vi "USB2XXXSPIW25Q32.vi"() -> ()   [LabVIEW 2010]
uses:
  PublicFiles/usb_device/USB2XXX.dll
panel:
  in  "pConfig":T1
  out "Read Data(Hex)":string
  in  "Read Data Count":i32=8
  in  "Start Addr(Hex)":u32 format="%x"
  in  "Write Data(Hex)":string="11 22 33 44 55 66 77 88"
  in  "Channel Index":i32(ring) items=["SPI1_CS0", "SPI2_CS0"]
  in  "Device Index":i32(ring) items=["0", "1", "2", "3", "4", "5"]
  out "Flag(T:Write;F:Read)":bool=TRUE
  in  "stop":bool
  in  "Read":bool
  in  "Write":bool
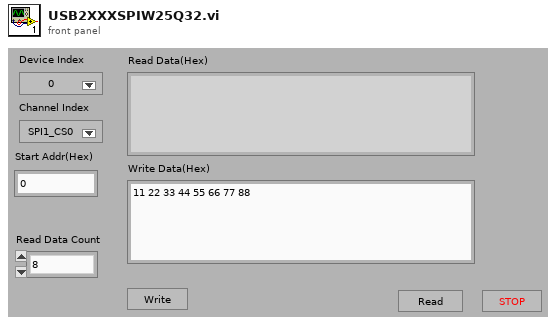
[diagram p1: front panel]
types:
  T1 = cluster{"Mode":i8, "Master":i8, "CPOL":i8, "CPHA":i8, "LSBFirst":i8, "SelPolarity":i8, "@dummy control@":i8, "@dummy control@":i8, "ClockSpeedHz":u32}
  T2 = enum16{"Init", "Write", "Read", "Idel", "Close", "Erase"}
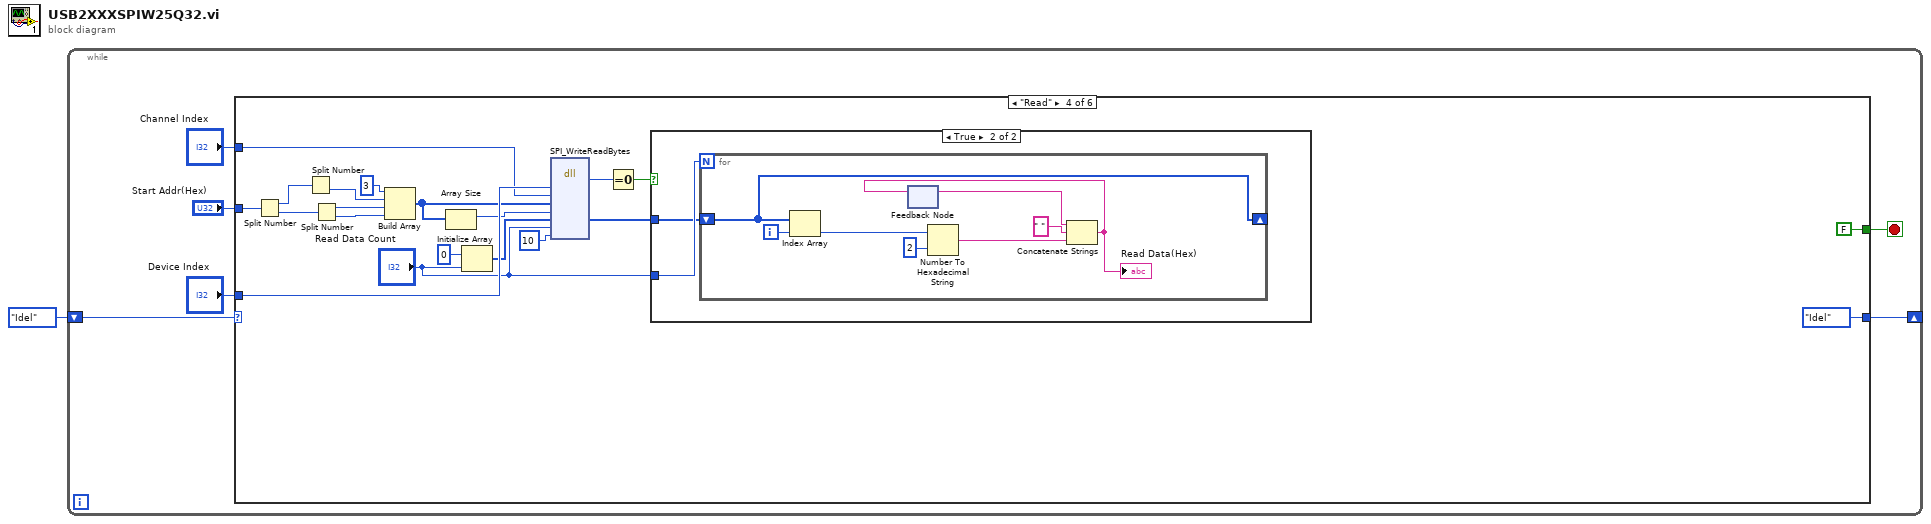
[diagram p0: block diagram]
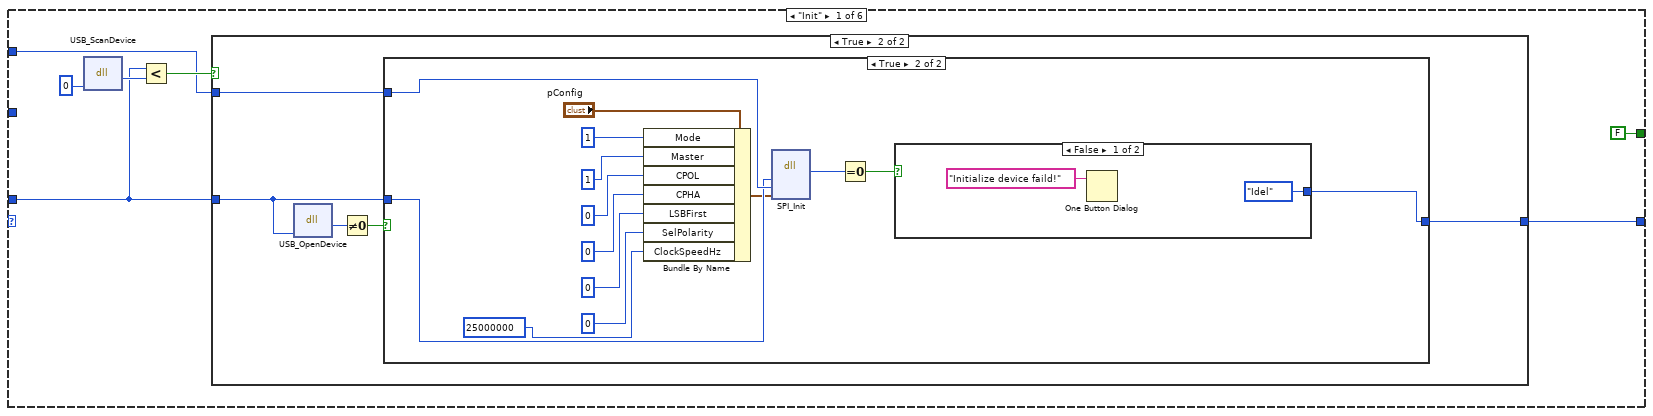
[diagram p2: hidden frame]
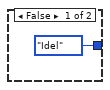
[diagram p3: hidden frame]
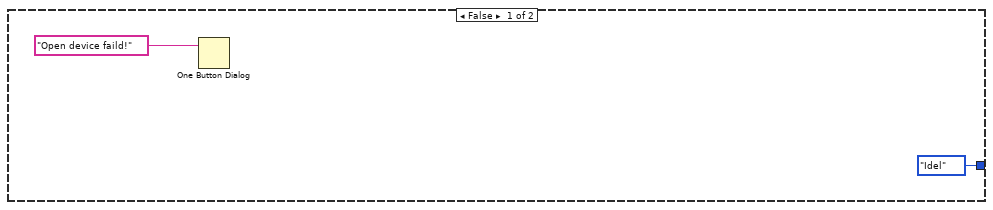
[diagram p4: hidden frame]
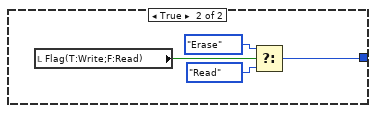
[diagram p5: hidden frame]
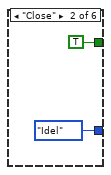
[diagram p6: hidden frame]
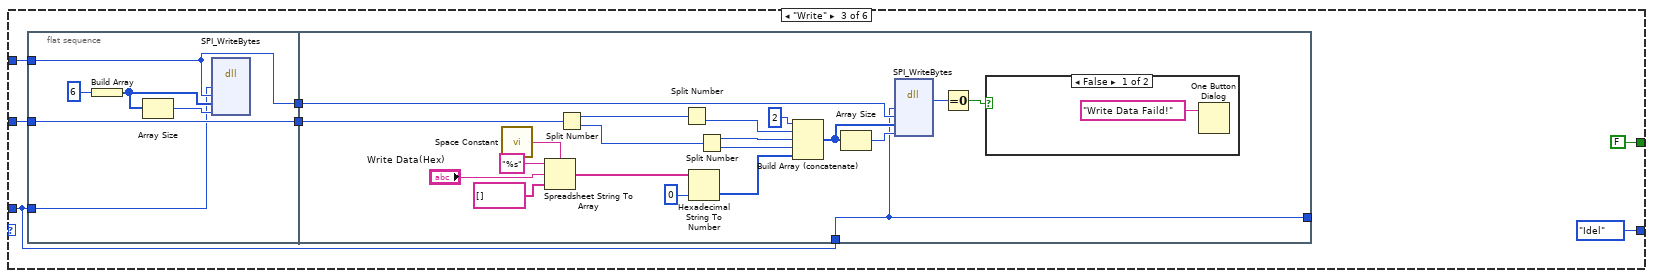
[diagram p7: hidden frame]
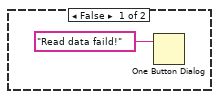
[diagram p9: hidden frame]
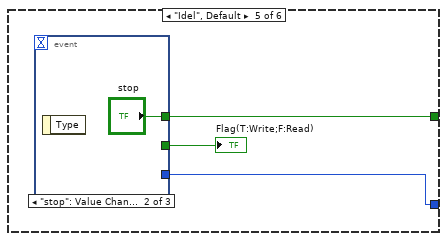
[diagram p10: hidden frame]
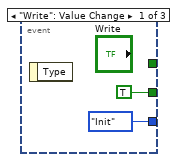
[diagram p11: hidden frame]
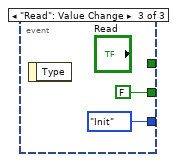
[diagram p12: hidden frame]
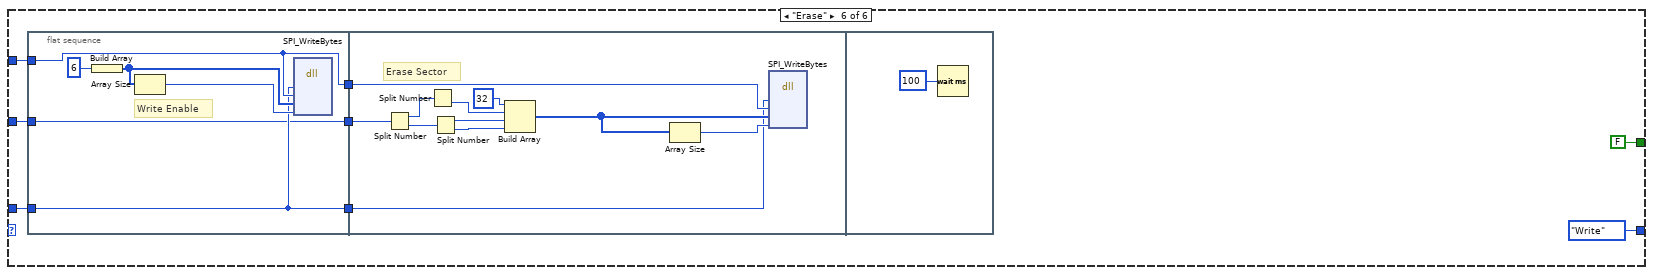
[diagram p13: hidden frame]
diagram:
  n1 = while {
    shift-right: [w6] -> _
    shift-left: T2."Idel" ("Enum") -> [w7]
    stop <- w2 stop-if-true
    n2 = case shown="\"Read\"" w7 {
      tunnel: [w11 T2."Idel" ("Enum") T2."Idel" ("Enum") T2."Idel" ("Enum") w110 T2."Write" ("Enum")] -> w6
      tunnel: "Device Index" -> [w8 _ w45 w87 _ w124]
      tunnel: "Channel Index" -> [w10 _ w50 w86 _ w123]
      tunnel: "Start Addr(Hex)" -> [_ _ w49 w89 _ w120]
      tunnel: [FALSE TRUE FALSE FALSE w111 FALSE] -> w2
      frame "Init" {
        n3 = dll-call lib="F:/OtherWork/STM32/USB2XXX_Example/trunk/Labview/PublicFiles/usb_device/USB2XXX.*" fn="USB_ScanDevice"("pDevNum"=0) -> (w13:i32)  [unwired: 4 in, 2 out]
        n4 = Less?(x=w8, y=w13) -> (x < y?=w12:bool)
        n5 = case shown="True" w12 {
          tunnel: w8 -> [_ w16]
          tunnel: w10 -> [_ w18]
          tunnel: [T2."Idel" ("Enum") w17] -> w11
          frame False {
          }
          frame True {
            n6 = dll-call lib="F:/OtherWork/STM32/USB2XXX_Example/trunk/Labview/PublicFiles/usb_device/USB2XXX.*" fn="USB_OpenDevice"("DevIndex"=w16) -> (w20:u8)  [unwired: 4 in, 2 out]
            n7 = Not Equal To 0?(x=w20) -> (x != 0?=w19:bool)
            n8 = case shown="True" w19 {
              tunnel: w18 -> [_ w34]
              tunnel: w16 -> [_ w33]
              tunnel: [T2."Idel" ("Enum") w35] -> w17
              frame False {
                n9 = One Button Dialog(message="Open device faild!") -> ()  [unwired: 1 in, 1 out]
              }
              frame True {
                n10 = Bundle By Name(cluster="pConfig", "Mode"=i8 1, "Master"=i8 1, "CPOL"=i8 0, "CPHA"=i8 0, "LSBFirst"=i8 0, "SelPolarity"=i8 0, "ClockSpeedHz"=u32 25000000) -> (w32:T1)
                n11 = dll-call lib="F:/OtherWork/STM32/USB2XXX_Example/trunk/Labview/PublicFiles/usb_device/USB2XXX.*" fn="SPI_Init"("DevIndex"=w33, "SPIIndex"=w34, "pConfig"=w32) -> (w31:i32)  [unwired: 6 in, 2 out]
                n12 = Equal To 0?(x=w31) -> (x = 0?=w36:bool)
                n13 = case shown="False" w36 {
                  tunnel: [T2."Idel" ("Enum") w41] -> w35
                  frame False {
                    n14 = One Button Dialog(message="Initialize device faild!") -> ()  [unwired: 1 in, 1 out]
                  }
                  frame True {
                    n15 = local read "Flag(T:Write;F:Read)"() -> (w42:bool)
                    n16 = Select(t=T2."Erase" ("Enum"), s=w42, f=T2."Read" ("Enum")) -> (s? t:f=w41:T2)
                  }
                }
              }
            }
          }
        }
      }
      frame "Close" {
      }
      frame "Write" {
        n17 = flat-sequence {
          tunnel: w45 -> [w52]
          tunnel: w50 -> [w53]
          tunnel: w49 -> [w54]
          tunnel: [w54] -> w48
          tunnel: [w53] -> w47
          tunnel: w48 -> [w60]
          tunnel: w47 -> [w59]
          tunnel: [w58] -> _
          tunnel: w45 -> [w58]
          frame #0 {
            n18 = Build Array(u8 6) -> (w56:u8[])
            n19 = Array Size(array=w56) -> (size(s)=w55:i32)
            n20 = dll-call lib="F:/OtherWork/STM32/USB2XXX_Example/trunk/Labview/PublicFiles/usb_device/USB2XXX.*" fn="SPI_WriteBytes"("DevIndex"=w52, "SPIIndex"=w53, "pWriteData"=w56, "WriteLen"=w55) -> ()  [unwired: 8 in, 2 out]
          }
          frame #1 {
            n21 = call <vilib>:"Space Constant.vi"() -> ("String"=w65:string)
            n22 = Spreadsheet String To Array(delimiter (Tab)=w65, format string="%s", spreadsheet string="Write Data(Hex)", array type (2D Dbl)=string[] []) -> (array=w62:string[])
            n23 = Split Number(x=w60) -> (hi(x)=w69:u16, lo(x)=w70:u16)
            n24 = Split Number(x=w69) -> (lo(x)=w71:u8)  [unwired: 1 out]
            n25 = Hexadecimal String To Number(string=w62, default (0uL)=u8 0 ("default (0 U32)")) -> (number=w74:u8[])  [unwired: 1 in, 1 out]
            n26 = Split Number(x=w70) -> (hi(x)=w72:u8, lo(x)=w73:u8)
            n27 = Build Array (concatenate)(u8 2, w71, w72, w73, w74) -> (w77:u8[])
            n28 = Array Size(array=w77) -> (size(s)=w75:i32)
            n29 = dll-call lib="F:/OtherWork/STM32/USB2XXX_Example/trunk/Labview/PublicFiles/usb_device/USB2XXX.*" fn="SPI_WriteBytes"("DevIndex"=w58, "SPIIndex"=w59, "pWriteData"=w77, "WriteLen"=w75) -> (w76:i32)  [unwired: 7 in, 2 out]
            n30 = Equal To 0?(x=w76) -> (x = 0?=w67:bool)
            n31 = case shown="False" w67 {
              frame False {
                n32 = One Button Dialog(message="Write Data Faild!") -> ()  [unwired: 1 in, 1 out]
              }
              frame True {
              }
            }
          }
        }
      }
      frame "Read" {
        n33 = Split Number(x=w89) -> (hi(x)=w94:u16, lo(x)=w93:u16)
        n34 = Split Number(x=w94) -> (lo(x)=w92:u8)  [unwired: 1 out]
        n35 = Split Number(x=w93) -> (hi(x)=w91:u8, lo(x)=w90:u8)
        n36 = Build Array(u8 3, w92, w91, w90) -> (w85:u8[])
        n37 = Array Size(array=w85) -> (size(s)=w84:i32)
        n38 = Initialize Array(u8 0 ("element"), "Read Data Count") -> (w83:u8[])
        n39 = dll-call lib="F:/OtherWork/STM32/USB2XXX_Example/trunk/Labview/PublicFiles/usb_device/USB2XXX.*" fn="SPI_WriteReadBytes"("DevIndex"=w87, "SPIIndex"=w86, "pWriteData"=w85, "WriteLen"=w84, "pReadData"=w83, "ReadLen"="Read Data Count", "IntervalTimeUs"=10 ("TimeOutMs")) -> (w88:i32, "pReadData"=w80:u8[])  [unwired: 9 in, 2 out]
        n40 = Equal To 0?(x=w88) -> (x = 0?=w97:bool)
        n41 = case shown="True" w97 {
          tunnel: "Read Data Count" -> [_ w101]
          tunnel: w80 -> [_ w100]
          frame False {
            n42 = One Button Dialog(message="Read data faild!") -> ()  [unwired: 1 in, 1 out]
          }
          frame True {
            n43 = for {
              N: w101 -> [_]
              shift-right: [w102] -> _
              shift-left: w100 -> [w102]
              i -> [w109]
              n44 = Index Array(array=w102, index=w109) -> (element=w108:u8)
              n45 = feedback #1() -> (w106:string)  [unwired: 1 in]
              n46 = Number To Hexadecimal String(1:i16 2 ("width (-)"), 2:w108) -> (0:w104:string)
              n47 = Concatenate Strings(w106, " " ("string"), w104) -> (w103:string)
              "Read Data(Hex)" <- w103
              n48 = feedback-in #1(w103) -> ()
            }
          }
        }
      }
      frame "Idel", Default {
        n49 = event shown="[1] \"stop\": Value Change" {
          selector: _ -> [_ _ _]
          dyn-events: _ -> [_ _ _]
          timeout: _ -> [_ _ _]
          tunnel: [TRUE _ FALSE] -> w112
          tunnel: [_ "stop" _] -> w111
          tunnel: [T2."Init" ("Enum") _ T2."Init" ("Enum")] -> w110
          event "Write": Value Change {
            n50 = event-data() -> ()  [unwired: 1 in, 1 out]
          }
          event "stop": Value Change {
            n51 = event-data() -> ()  [unwired: 1 in, 1 out]
          }
          event "Read": Value Change {
            n52 = event-data() -> ()  [unwired: 1 in, 1 out]
          }
        }
        "Flag(T:Write;F:Read)" <- w112
      }
      frame "Erase" {
        n53 = flat-sequence {
          tunnel: w124 -> [w127]
          tunnel: w123 -> [w128]
          tunnel: [w128] -> w122
          tunnel: [w127] -> w121
          tunnel: w120 -> [w126]
          tunnel: [w126] -> w119
          tunnel: w122 -> [w139]
          tunnel: w121 -> [w138]
          tunnel: w119 -> [w137]
          frame #0 {
            # "Write Enable"
            n54 = Build Array(u8 6) -> (w130:u8[])
            n55 = Array Size(array=w130) -> (size(s)=w129:i32)
            n56 = dll-call lib="F:/OtherWork/STM32/USB2XXX_Example/trunk/Labview/PublicFiles/usb_device/USB2XXX.*" fn="SPI_WriteBytes"("DevIndex"=w127, "SPIIndex"=w128, "pWriteData"=w130, "WriteLen"=w129) -> ()  [unwired: 8 in, 2 out]
          }
          frame #1 {
            # "Erase Sector"
            n57 = Split Number(x=w137) -> (hi(x)=w136:u16, lo(x)=w135:u16)
            n58 = Split Number(x=w136) -> (lo(x)=w134:u8)  [unwired: 1 out]
            n59 = Split Number(x=w135) -> (hi(x)=w133:u8, lo(x)=w132:u8)
            n60 = Build Array(u8 32, w134, w133, w132) -> (w141:u8[])
            n61 = Array Size(array=w141) -> (size(s)=w140:i32)
            n62 = dll-call lib="F:/OtherWork/STM32/USB2XXX_Example/trunk/Labview/PublicFiles/usb_device/USB2XXX.*" fn="SPI_WriteBytes"("DevIndex"=w138, "SPIIndex"=w139, "pWriteData"=w141, "WriteLen"=w140) -> ()  [unwired: 8 in, 2 out]
          }
          frame #2 {
            n63 = Wait (ms)(milliseconds to wait=u32 100) -> ()  [unwired: 1 out]
          }
        }
      }
    }
  }
